vi "init_daq_ai_di.vi"(10 "Sample Rate":dbl) -> (0 "error out":errorcluster, 2 "DI Out":refnum<k21>, 3 "AI Out":refnum<k21>, 5 "Actual Sample Rate":dbl=1000.0 format="%0.2f")   [LabVIEW 2015]
uses:
  <vilib>/DAQmx/create/channels.llb/DAQmx Create Channel (AI-Voltage-Basic).vi
  <vilib>/DAQmx/configure/timing.llb/DAQmx Timing (Sample Clock).vi
  <vilib>/DAQmx/create/channels.llb/DAQmx Create Channel (DI-Digital Input).vi
  <resource>/objmgr/daqmx.rc
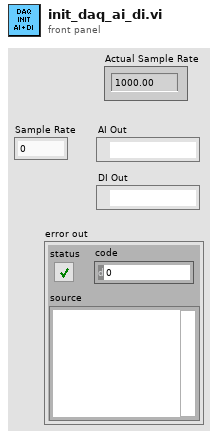
[diagram p1: front panel]
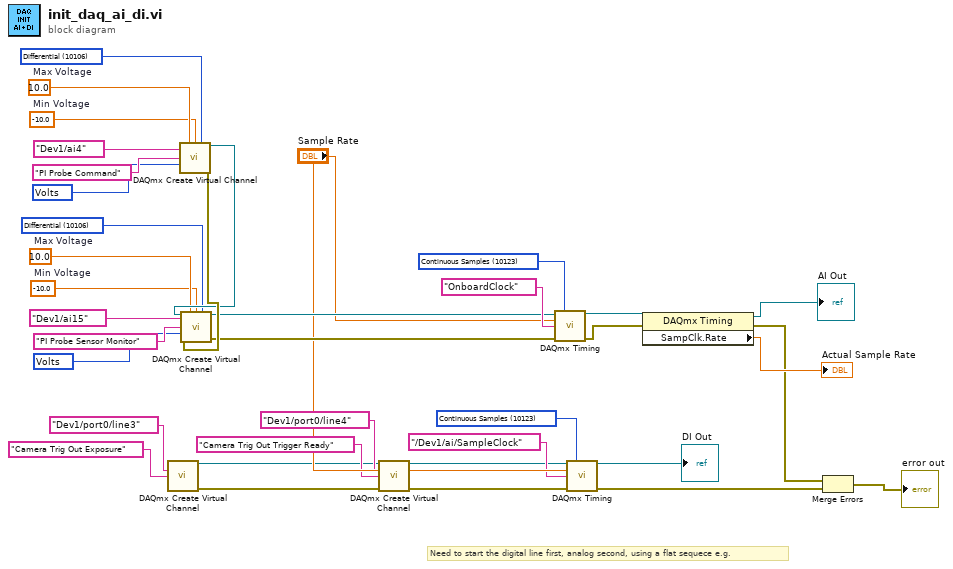
[diagram p0: block diagram]
diagram:
  w13 = 10123 items=["Finite Samples"=10178, "Continuous Samples"=10123, "Hardware Timed Single Point"=12522] ("sample mode")
  w20 = 10123 items=["Finite Samples"=10178, "Continuous Samples"=10123] ("sample mode")
  w34 = 10348 items=["Volts"=10348, "From Custom Scale"=10065] ("units")
  w33 = 10106 items=["default"=-1, "RSE"=10083, "NRSE"=10078, "Differential"=10106, "Pseudodifferential"=12529] ("input terminal configuration")
  w31 = -10.0  # Min Voltage
  w32 = 10.0  # Max Voltage
  w29 = 10348 items=["Volts"=10348, "From Custom Scale"=10065] ("units")
  w28 = 10106 items=["default"=-1, "RSE"=10083, "NRSE"=10078, "Differential"=10106, "Pseudodifferential"=12529] ("input terminal configuration")
  w26 = -10.0  # Min Voltage
  w27 = 10.0  # Max Voltage
  # "Need to start the digital line first, analog second, using a flat sequece e.g."
  n1 = call-poly <vilib>:"DAQmx Create Virtual Channel.vi"("lines"=tag "Dev1/port0/line3", "name to assign"="Camera Trig Out Exposure") -> ("task out"=w2:refnum<k21>, "error out"=w1:errorcluster)  [unwired: 12 in]
  n2 = call-poly <vilib>:"DAQmx Create Virtual Channel.vi"("maximum value"=w27, "minimum value"=w26, "input terminal configuration"=w28, "physical channels"=tag "Dev1/ai4", "name to assign"="PI Probe Command", "units"=w29) -> ("task out"=w36:refnum<k21>, "error out"=w37:errorcluster)  [unwired: 8 in]
  n3 = call-poly <vilib>:"DAQmx Create Virtual Channel.vi"("task in"=w36, "maximum value"=w32, "minimum value"=w31, "input terminal configuration"=w33, "physical channels"=tag "Dev1/ai15", "name to assign"="PI Probe Sensor Monitor", "units"=w34, "error in"=w37) -> ("task out"=w15:refnum<k21>, "error out"=w14:errorcluster)  [unwired: 6 in]
  n4 = call-poly <vilib>:"DAQmx Create Virtual Channel.vi"("task in"=w2, "lines"=tag "Dev1/port0/line4", "name to assign"="Camera Trig Out Trigger Ready", "error in"=w1) -> ("task out"=w4:refnum<k21>, "error out"=w3:errorcluster)  [unwired: 10 in]
  n5 = call-poly <vilib>:"DAQmx Timing.vi"("task/channels in"=w15, "sample mode"=w20, "rate"="Sample Rate", "source"=tag "OnboardClock" ("Sample Clock Source"), "error in"=w14) -> ("task out"=w25:refnum<k21>, "error out"=w24:errorcluster)  [unwired: 9 in]
  n6 = call-poly <vilib>:"DAQmx Timing.vi"("task/channels in"=w4, "sample mode"=w13, "rate"="Sample Rate", "source"=tag "/Dev1/ai/SampleClock", "error in"=w3) -> ("task out"=→"DI Out":refnum<k21>, "error out"=w9:errorcluster)  [unwired: 9 in]
  n7 = property class="DAQmx Timing"(reference=w25, error in=w24) -> (reference out=→"AI Out":refnum<k21>, error out=w8:errorcluster, "SampClk.Rate"=→"Actual Sample Rate":dbl)
  n8 = Merge Errors(w8, w9) -> (→"error out":errorcluster)
